vi "Initialize.vi"(8 "error in (no error)":errorcluster, 10 "Raw Record String":string, 11 "Record in":refnum<class "Record.lvclass">) -> (0 "error out":errorcluster, 1 "value 2":string, 2 "value":string, 3 "Record out":refnum<class "Record.lvclass">)   [LabVIEW 2019, in "Record.lvclass"]
uses:
  Record.lvclass
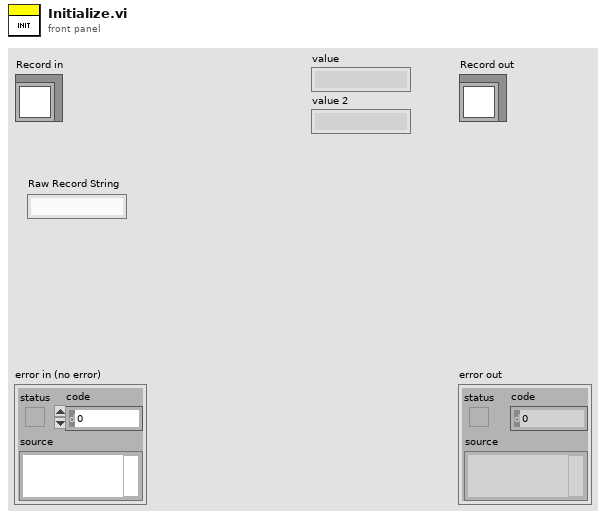
[diagram p1: front panel]
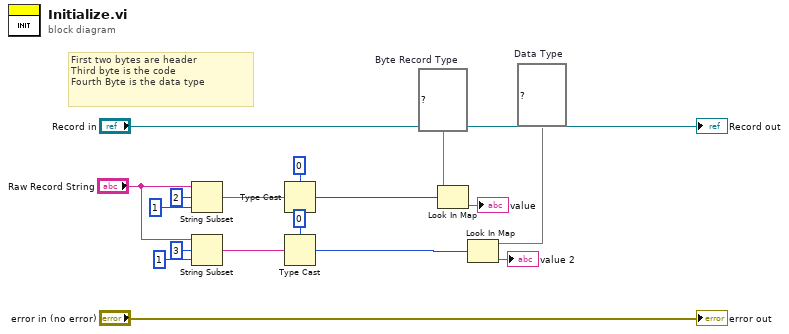
[diagram p0: block diagram]
diagram:
  w2 = map{i8, string} {0="No Data", 1="Bit Array", 2="Word", 3="Long", 5="Real", 6="String"}  # Data Type
  w11 = map{i32, string} {0="HEADER", 1="BGNLIB", 2="LIBNAME", 3="UNITS", 4="ENDLIB", 5="BGNSTR", 6="STRNAME", 7="ENDSTR", 8="BOUNDARY", 9="PATH", 10="SREF", 11="AREF", 12="TEXT", 13="LAYER", 14="DATATYPE", 15="WIDTH", 16="XY", 17="ENDEL", 18="SNAME", 19="COLROW", 21="NODE", 22="TEXTTYPE", 23="PRESENTATION", 25="STRING", 26="STRANS", 27="MAG", 28="ANGLE", 31="REFLIBS", 32="FONTS", 33="PATHTYPE", 34="GENERATIONS", 35="ATTRTABLE", 38="ELFLAGS", 42="NODETYPE", 43="PROPATTR", 44="PROPVALUE", 45="BOX", 46="BOXTYPE", 47="PLEX", 50="TAPENUM", 51="TAPECODE", 54="FORMAT", 55="MASK", 56="ENDMASKS"}  # Byte Record Type
  # "First two bytes are header\nThird byte is the code\nFourth Byte is the data type"
  n1 = String Subset(string="Raw Record String", offset (0)=2, length (rest)=1 ("length (rest)")) -> (substring=w13:string)
  n2 = String Subset(string="Raw Record String", offset (0)=3, length (rest)=1 ("length (rest)")) -> (substring=w4:string)
  n3 = Type Cast(type=i8 0 ("offset (0)"), x=w13) -> (*(type *) &x=w10:i8)
  n4 = Type Cast(type=i8 0 ("offset (0)"), x=w4) -> (*(type *) &x=w3:i8)
  n5 = Look In Map(map=w11, key=w10) -> (value=→"value":string)  [unwired: 1 in, 1 out]
  n6 = Look In Map(map=w2, key=w3) -> (value=→"value 2":string)  [unwired: 1 in, 1 out]
  "error out" <- "error in (no error)"
  "Record out" <- "Record in"
